vi "Result_Test.vi"(8 "error in (no error)":errorcluster caption="entrée d'erreur (pas d'erreur)", 11 "Get_Voltage en entrée":refnum<class "Read_Intensity_LED.lvclass">) -> (0 "error out":errorcluster caption="sortie d'erreur", 3 "Get_Voltage en sortie":refnum<class "Read_Intensity_LED.lvclass">)   [LabVIEW 2020, in "Library Test.lvlib" / "Read_Intensity_LED.lvclass"]
uses:
  Read_Intensity_LED.lvclass
  C:/Users/ngarcin/OneDrive - Altyor/Standard TB/Class/Test/Test (Default)/Test (Default).lvclass
  JSON API/JSON Value/Set from JSON string.vi
  Instrument/Instrument (Default)/Class Instrument (Default).lvclass
  JSON API/JSON Value/JSON Value.lvclass
  Read_Led_Analyser/Read_Led_Analyser.lvclass
  Read_Intensity_LED.lvclass/Read_Intensity_LED.ctl
  JSON API/Variant JSON/Variant JSON.lvlib
  JSON API/Get Polymorphic/JSON GetSet.lvlib
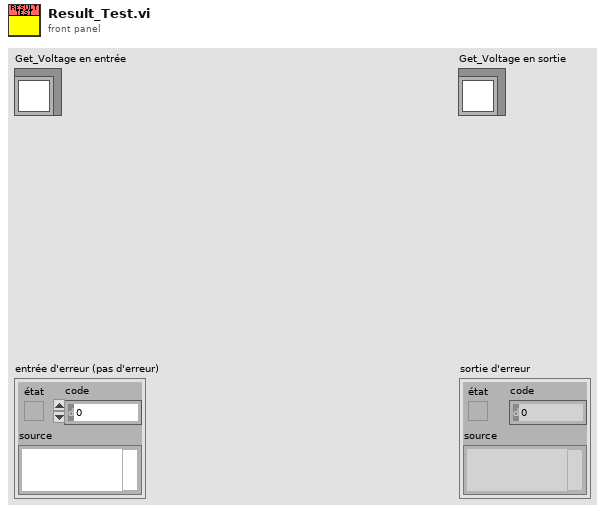
[diagram p1: front panel]
types:
  T1 = cluster{"Hue":dbl, "Saturation":u32, "Intensity":u32}
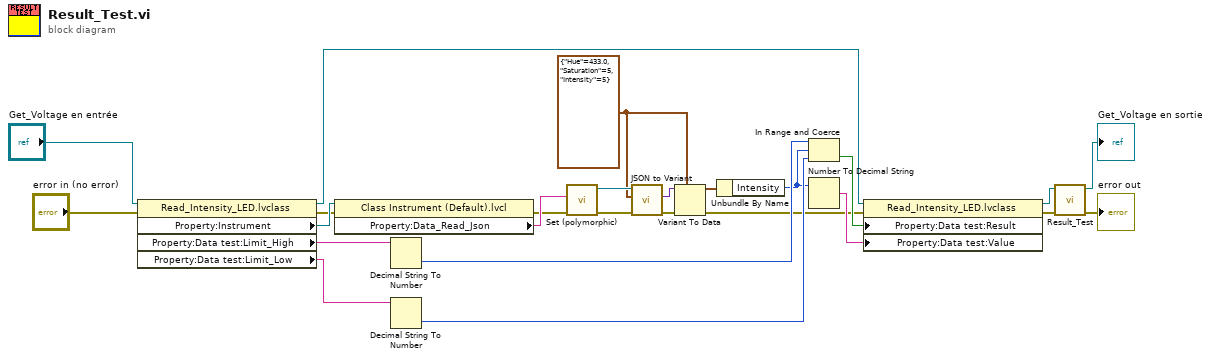
[diagram p0: block diagram]
diagram:
  w17 = T1 {"Hue"=433.0, "Saturation"=5, "Intensity"=5} ("Parameter")
  n1 = property class="Read_Intensity_LED.lvclass"(reference="Get_Voltage en entrée", error in="error in (no error)") -> (reference out=w15:refnum<class "Read_Intensity_LED.lvclass">, error out=w2:errorcluster, "Property:Instrument"=w4:refnum<class "Class Instrument (Default).lvclass">, "Property:Data test:Limit_High"=w14:string, "Property:Data test:Limit_Low"=w13:string)
  n2 = property class="Class Instrument (Default).lvcl"(reference=w4, error in=w2) -> (error out=w1:errorcluster, "Property:Data_Read_Json"=w3:string)  [unwired: 1 out]
  n3 = Decimal String To Number(string=w14) -> (number=w12:i32)  [unwired: 2 in, 1 out]
  n4 = Decimal String To Number(string=w13) -> (number=w11:i32)  [unwired: 2 in, 1 out]
  n5 = call-poly "Set (polymorphic).vi"("error in (no error)"=w1, "JSON stream"=w3) -> ("error out"=w21:errorcluster, "JSON Value out"=w19:refnum<class "JSON Value.lvclass">)  [unwired: 7 in, 1 out]
  n6 = call "JSON to Variant.vi"("error in (no error)"=w21, "Variant (Data Type)"=w17, "JSON Value"=w19) -> ("error out"=w20:errorcluster, "Variant out"=w18:variant)  [unwired: 7 in]
  n7 = Variant To Data(error in=w20, type=w17, Variant=w18) -> (data=w16:T1, error out=w7:errorcluster)
  n8 = Unbundle By Name(w16) -> ("Intensity"=w9:u32)
  n9 = In Range and Coerce(upper limit=w12, x=w9, lower limit=w11) -> (In Range?=w10:bool)  [unwired: 1 out]
  n10 = Number To Decimal String(number=w9) -> (decimal integer string=w8:string)  [unwired: 1 in]
  n11 = property class="Read_Intensity_LED.lvclass"(reference=w15, error in=w7, "Property:Data test:Result"=w10, "Property:Data test:Value"=w8) -> (reference out=w6:refnum<class "Read_Intensity_LED.lvclass">, error out=w5:errorcluster)
  n12 = call-parent "Result_Test.vi"("error in (no error)"=w5, "Get_Voltage en entrée"=w6) -> ("error out"=→"error out":errorcluster, "Get_Voltage en sortie"=→"Get_Voltage en sortie":refnum<class "Read_Intensity_LED.lvclass">)  [unwired: 8 in]
